vi "engine mappings UI.vi"() -> ()   [LabVIEW 2013, in "PL Framework Configuration Tool.lvlib" / "Engine Mappings.lvclass"]
uses:
  Engine Mappings.lvclass
  <vilib>/NI/CEF/CEF_TreeControl/Controls/EventCluster.ctl
  <vilib>/NI/CEF/CEF_TreeControl/NISE_CEF_TreeControl.lvlib
  <vilib>/NI/Module Execution Interface/Engine Configuration/engine configuration.lvclass
  <vilib>/NI/Tag Bus/tag/tag descriptor.lvclass
  Engine Parent/Engine Parent Editor Node.lvclass
  <vilib>/NI/CEF/CEF_TreeControl/Node/NodeRef.ctl
  <vilib>/NI/CEF/CEF_TreeControl/Node/NISE_CEF_Node.lvclass
  <vilib>/NI/Tools/Keyed Array/KeyedArray.ctl
  <vilib>/NI/Tools/Keyed Array/Tools_KeyedArray.lvlib
  <vilib>/NI/AMC/Message.ctl
  <vilib>/NI/AMC/AMC.lvlib
  <vilib>/NI/AMC/Message Queue.ctl
  <vilib>/NI/CEF/CEF_TreeControl/Node/UserEventRef.ctl
panel:
  in  "channels":i32(listbox)
  in  "main queue":T1
  in  "node ref":T2
  in  "Tags":i32(listbox)
  in  "user event":T3
  in  "unmap":bool
  in  "map":bool
  in  "Mappings":i32(listbox)
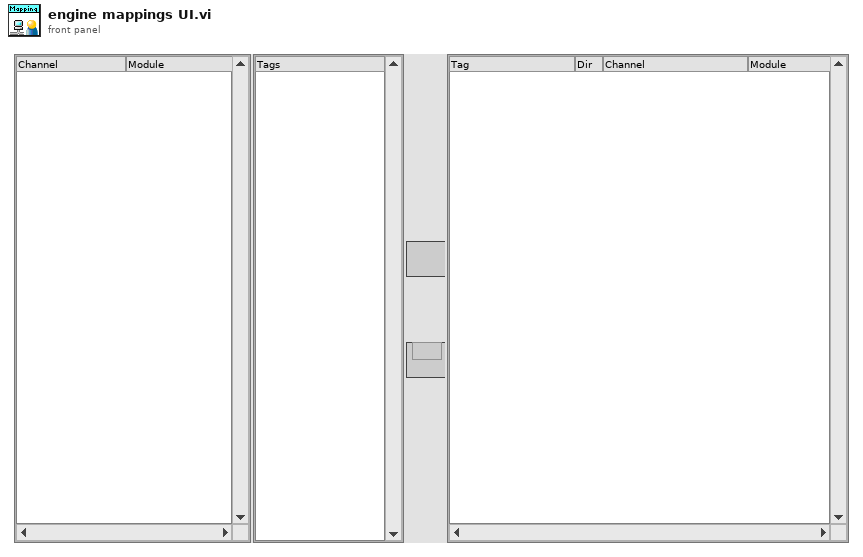
[diagram p1: front panel]
types:
  T1 = typedef "AMC.lvlib/Message Queue.ctl" = refnum<queue>
  T2 = typedef "NISE_CEF_Node.lvclass/NodeRef.ctl" = refnum<data-value>
  T3 = typedef "NISE_CEF_Node.lvclass/UserEventRef.ctl" = refnum<user-event>
  T4 = typedef "NISE_CEF_TreeControl.lvlib/EventCluster.ctl" = cluster{"command":string, "data":string}
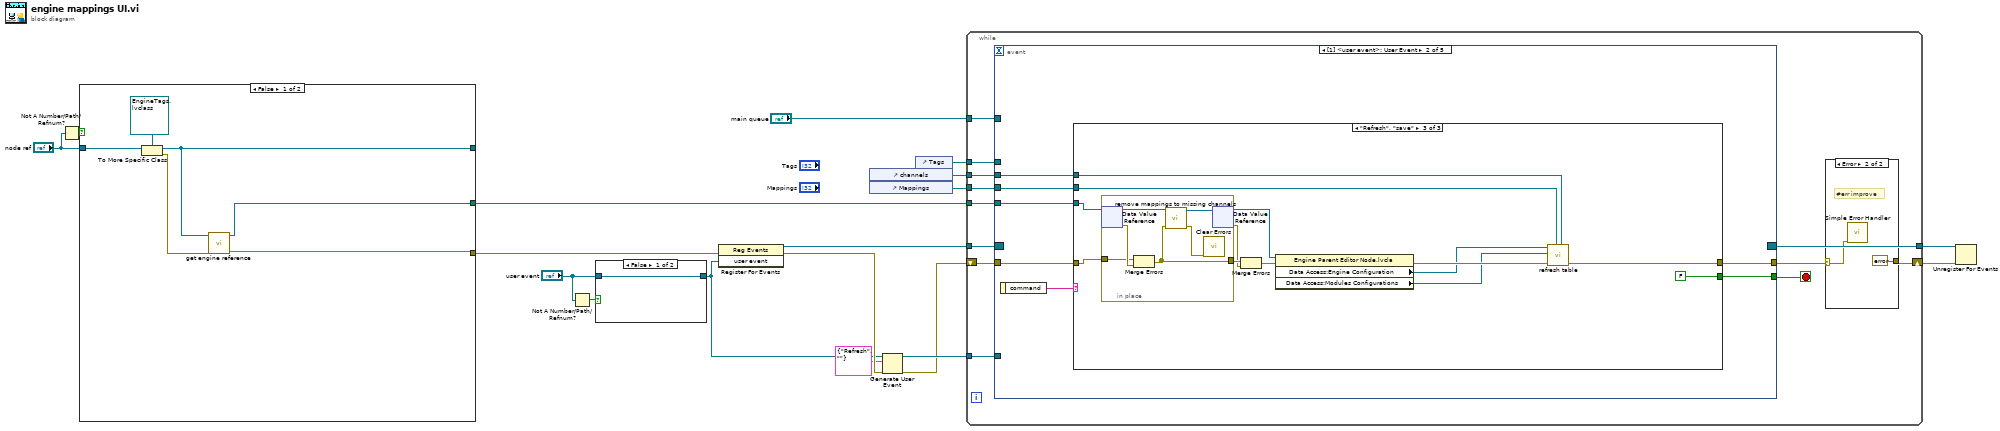
[diagram p0: block diagram]
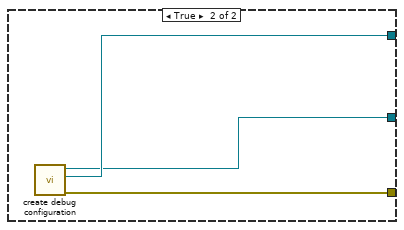
[diagram p2: hidden frame]
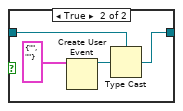
[diagram p3: hidden frame]
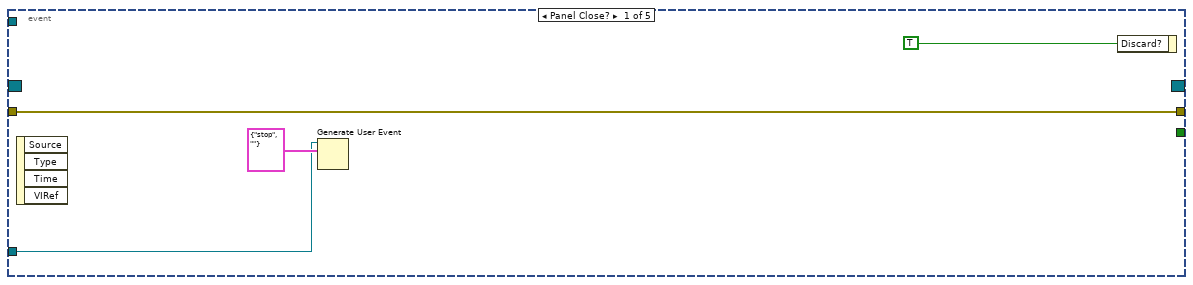
[diagram p5: hidden frame]
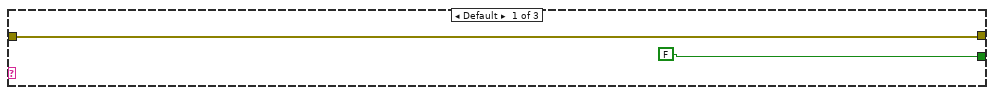
[diagram p6: hidden frame]
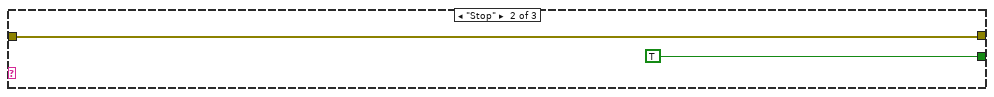
[diagram p7: hidden frame]
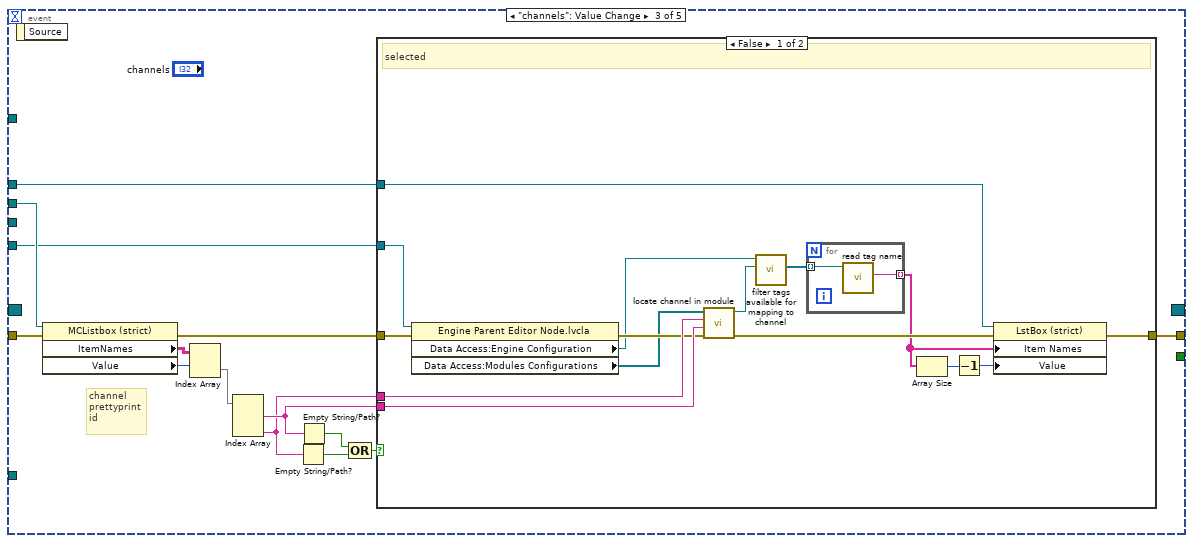
[diagram p8: hidden frame]
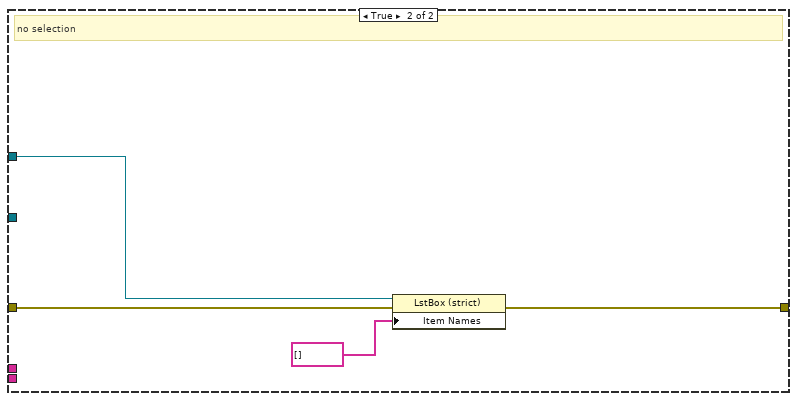
[diagram p9: hidden frame]
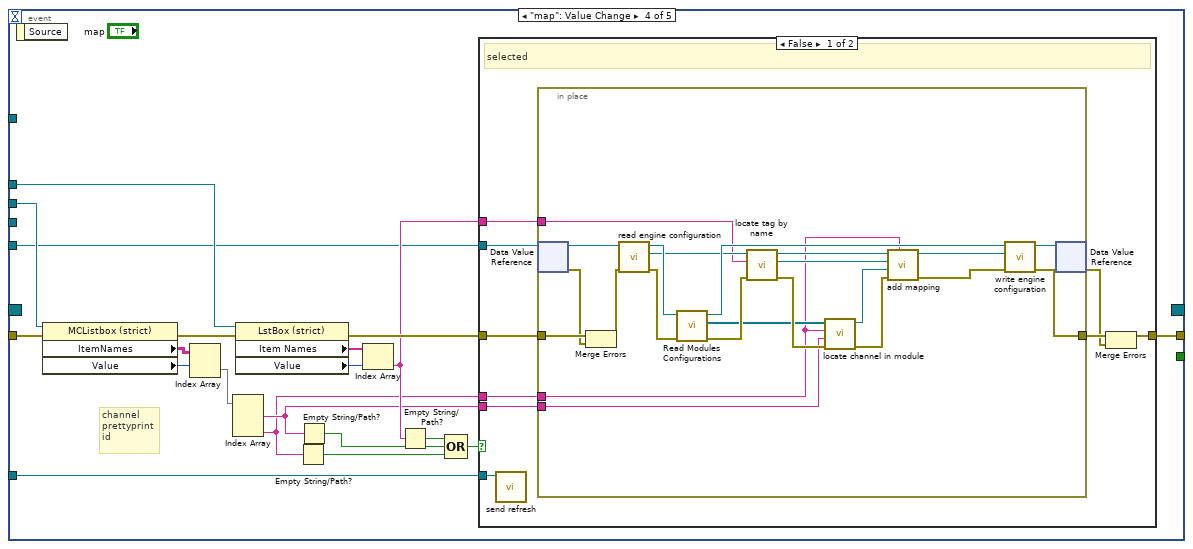
[diagram p10: hidden frame]
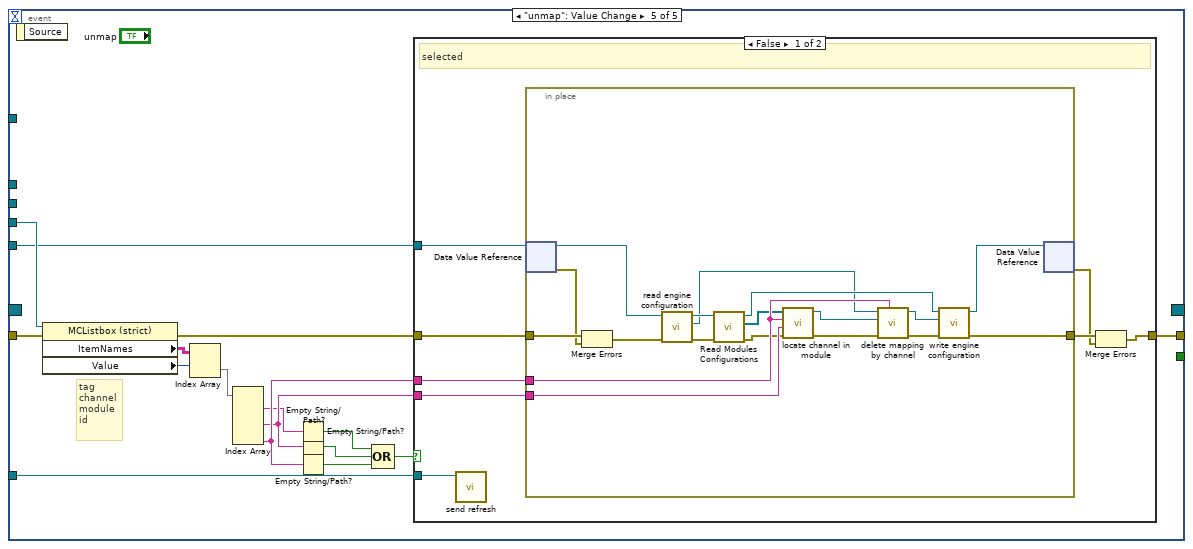
[diagram p12: hidden frame]
diagram:
  n1 = Not A Number/Path/Refnum?(number/path/refnum="node ref") -> (NaN/Path/Refnum?=w9:bool)
  n2 = case shown="False" w9 {
    tunnel: [w21 w27] -> _
    tunnel: [w22 w26] -> w1
    tunnel: [w20 w25] -> w13
    tunnel: "node ref" -> [w19 _]
    frame False {
      n3 = To More Specific Class(target class=refnum<data-value> refnum ("data value reference"), reference=w19) -> (specific class reference=w21:refnum<data-value>, error out=w23:errorcluster)  [unwired: 1 in]
      n4 = call "get engine reference.vi"("error in"=w23, "engine mappings"=w21) -> ("error out"=w22:errorcluster, "engine reference"=w20:refnum<data-value>)  [unwired: 8 in]
    }
    frame True {
      n5 = call "create debug configuration.vi"() -> ("error out"=w26:errorcluster, "mapping dvr"=w27:refnum<data-value>, "engine dvr"=w25:refnum<data-value>)  [unwired: 9 in]
    }
  }
  n6 = Not A Number/Path/Refnum?(number/path/refnum="user event") -> (NaN/Path/Refnum?=w11:bool)
  n7 = case shown="False" w11 {
    tunnel: [w28 w29] -> w8
    tunnel: "user event" -> [w28 w30]
    frame False {
    }
    frame True {
      n8 = Create User Event(user event datatype=T4 {"command"="", "data"=""} ("event data")) -> (user event=w31:refnum<user-event>)  [unwired: 1 in, 1 out]
      n9 = Type Cast(type=w30, x=w31) -> (*(type *) &x=w29:T3)
    }
  }
  n10 = register-events(error in=w1, w8) -> (reference out=w17:refnum<event-registration>, error out=w14:errorcluster)  [unwired: 1 in]
  n11 = control-ref of="channels"() -> (w3:refnum<vi>)
  n12 = control-ref of="Mappings"() -> (w2:refnum<vi>)
  n13 = Generate User Event(user event=w8, event data cluster=T4 {"command"="Refresh", "data"=""} ("event data"), error in=w14) -> (user event out=w7:T3, error out=w6:errorcluster)  [unwired: 1 in]
  n14 = control-ref of="Tags"() -> (w4:refnum<vi>)
  n15 = while {
    tunnel: "main queue" -> [w44]
    tunnel: w17 -> [w43]
    tunnel: [w42] -> w16
    shift-right: [w40] -> w15
    shift-left: w6 -> [w39]
    tunnel: w13 -> [w38]
    tunnel: w7 -> [w36]
    tunnel: w4 -> [w35]
    tunnel: w3 -> [w34]
    tunnel: w2 -> [w33]
    stop <- w41 stop-if-true
    n16 = event shown="[1] <user event>: User Event" {
      selector: w43 -> [_ _ _ _ _]
      dyn-events: [_ _ _ _ _] -> w42
      timeout: _ -> [_ _ _ _ _]
      tunnel: w44 -> [_ _ _ _ _]
      tunnel: [_ w55 _ _ _] -> w41
      tunnel: w39 -> [w51 w58 w95 w136 w184]
      tunnel: [w51 w57 w86 w122 w177] -> w37
      tunnel: w38 -> [_ w56 w82 w117 w169]
      tunnel: w36 -> [w49 _ _ w121 w176]
      tunnel: w35 -> [_ _ w83 w135 _]
      tunnel: w34 -> [_ w53 w93 w133 _]
      tunnel: w33 -> [_ w52 _ _ w175]
      event Panel Close? {
        n17 = event-data() -> ()  [unwired: 1 in, 4 out]
        n18 = Generate User Event(user event=w49, event data cluster=T4 {"command"="stop", "data"=""} ("event data")) -> ()  [unwired: 2 in, 2 out]
        n19 = event-data("Discard?"=TRUE) -> ()  [unwired: 1 in, 1 out]
      }
      event User Event {
        n20 = event-data() -> ("command"=w54:string)  [unwired: 1 in]
        n21 = case shown="\"Refresh\", \"save\"" w54 {
          tunnel: w58 -> [w60 w62 w66]
          tunnel: [w60 w62 w74] -> w57
          tunnel: w56 -> [_ _ w68]
          tunnel: [FALSE TRUE FALSE] -> w55
          tunnel: w53 -> [_ _ w73]
          tunnel: w52 -> [_ _ w72]
          frame Default {
          }
          frame "Stop" {
          }
          frame "Refresh", "save" {
            n22 = in-place {
              in-place-border: w66 -> [w80]
              in-place-border: [w77] -> w65
              n23 = in-place-dvr #1(w68) -> (w79:refnum<class "Engine Parent Editor Node.lvclass">, w81:errorcluster)
              n24 = Merge Errors(w80, w81) -> (w77:errorcluster)
              n25 = call "remove mappings to missing channels.vi"("error in"=w77, "Engine Parent Editor Node in"=w79) -> ("error out"=w76:errorcluster, "Engine Parent Editor Node out"=w78:refnum<class "Engine Parent Editor Node.lvclass">)  [unwired: 8 in]
              n26 = call <vilib>:"Clear Errors.vi"("error in (no error)"=w76) -> ()  [unwired: 6 in, 1 out]
              n27 = in-place-dvr #1(w78) -> (w67:refnum<data-value>, w64:errorcluster)
            }
            n28 = Merge Errors(w65, w64) -> (w63:errorcluster)
            n29 = property class="Engine Parent Editor Node.lvcla"(reference=w67, error in=w63) -> (error out=w71:errorcluster, "Data Access:Engine Configuration"=w70:refnum<class "engine configuration.lvclass">, "Data Access:Modules Configurations"=w69:refnum<class "TBM module configuration.lvclass">[])  [unwired: 1 out]
            n30 = call "refresh table.vi"("channels ref"=w73, "Mappings"=w72, "error in"=w71, "Modules Configurations"=w69, "engine configuration in"=w70) -> ("error out"=w74:errorcluster)  [unwired: 6 in]
          }
        }
      }
      event "channels": Value Change {
        # "channel\nprettyprint\nid"
        n31 = event-data() -> ()  [unwired: 1 in, 1 out]
        n32 = property class="MCListbox (strict)"(reference=w93, error in=w95) -> (error out=w94:errorcluster, "ItemNames"=w91:string[][], "Value"=w92:i32)  [unwired: 1 out]
        n33 = Index Array(array=w91, index (row)=w92) -> (element=w90:string[])  [unwired: 1 in]
        n34 = Index Array(array=w90) -> (element #1=w85:string, element #3=w84:string)  [unwired: 3 in, 1 out]
        n35 = Empty String/Path?(string/path=w84) -> (empty?=w89:bool)
        n36 = Empty String/Path?(string/path=w85) -> (empty?=w88:bool)
        n37 = Compound Arithmetic op=OR(w88, w89) -> (w87:bool)
        n38 = case shown="False" w87 {
          tunnel: w94 -> [w110 w116]
          tunnel: [w105 w115] -> w86
          tunnel: w85 -> [w109 _]
          tunnel: w84 -> [w108 _]
          tunnel: w83 -> [w106 w114]
          tunnel: w82 -> [w99 _]
          frame False {
            # "selected"
            n39 = property class="Engine Parent Editor Node.lvcla"(reference=w99, error in=w110) -> (error out=w98:errorcluster, "Data Access:Engine Configuration"=w96:refnum<class "engine configuration.lvclass">, "Data Access:Modules Configurations"=w97:refnum<class "TBM module configuration.lvclass">[])  [unwired: 1 out]
            n40 = call "locate channel in module.vi"("error in"=w98, "channel name"=w109, "instance id"=w108, "Modules Configurations"=w97) -> ("error out"=w104:errorcluster, "channel"=w107:refnum<class "TBM channel.lvclass">)  [unwired: 6 in]
            n41 = call <vilib>:"filter tags available for mapping to channel.vi"("channel to map to"=w107, "engine configuration in"=w96) -> ("filtered tags"=w103:refnum<class "tag descriptor.lvclass">[])  [unwired: 8 in, 1 out]
            n42 = for {
              tunnel: w103 -> [w112] mode=indexing
              tunnel: [w111] -> w102 mode=indexing
              n43 = call <vilib>:"read tag name.vi"("system tag in"=w112) -> ("name"=w111:string)  [unwired: 8 in, 2 out]
            }
            n44 = Array Size(array=w102) -> (size(s)=w101:i32)
            n45 = Decrement(x=w101) -> (x-1=w100:i32)
            n46 = property class="LstBox (strict)"(reference=w106, error in=w104, "Item Names"=w102, "Value"=w100) -> (error out=w105:errorcluster)  [unwired: 1 out]
          }
          frame True {
            # "no selection"
            n47 = property class="LstBox (strict)"(reference=w114, error in=w116, "Item Names"=string[] []) -> (error out=w115:errorcluster)  [unwired: 1 out]
          }
        }
      }
      event "map": Value Change {
        # "channel\nprettyprint\nid"
        n48 = event-data() -> ()  [unwired: 1 in, 1 out]
        n49 = property class="MCListbox (strict)"(reference=w133, error in=w136) -> (error out=w134:errorcluster, "ItemNames"=w131:string[][], "Value"=w132:i32)  [unwired: 1 out]
        n50 = Index Array(array=w131, index (row)=w132) -> (element=w128:string[])  [unwired: 1 in]
        n51 = Index Array(array=w128) -> (element #1=w119:string, element #3=w118:string)  [unwired: 3 in, 1 out]
        n52 = property class="LstBox (strict)"(reference=w135, error in=w134) -> (error out=w123:errorcluster, "Item Names"=w130:string[], "Value"=w129:i32)  [unwired: 1 out]
        n53 = Empty String/Path?(string/path=w118) -> (empty?=w127:bool)
        n54 = Empty String/Path?(string/path=w119) -> (empty?=w126:bool)
        n55 = Index Array(array=w130, index=w129) -> (element=w120:string)
        n56 = Empty String/Path?(string/path=w120) -> (empty?=w125:bool)
        n57 = Compound Arithmetic op=OR(w125, w126, w127) -> (w124:bool)
        n58 = case shown="False" w124 {
          tunnel: w123 -> [w144 w168]
          tunnel: [w142 w168] -> w122
          tunnel: w121 -> [w145 _]
          tunnel: w120 -> [w139 _]
          tunnel: w119 -> [w137 _]
          tunnel: w118 -> [w138 _]
          tunnel: w117 -> [w140 _]
          frame False {
            # "selected"
            n59 = call "send refresh.vi"("User Event in"=w145) -> ()  [unwired: 11 in]
            n60 = in-place {
              in-place-border: w144 -> [w167]
              in-place-border: [w162] -> w143
              in-place-border: w139 -> [w156]
              in-place-border: w138 -> [w146]
              in-place-border: w137 -> [w152]
              n61 = in-place-dvr #2(w140) -> (w159:refnum<class "Engine Parent Editor Node.lvclass">, w166:errorcluster)
              n62 = Merge Errors(w167, w166) -> (w165:errorcluster)
              n63 = call "read engine configuration.vi"("error in"=w165, "Engine Parent Editor Node in"=w159) -> ("error out"=w164:errorcluster, "engine configuration"=w158:refnum<class "engine configuration.lvclass">, "Engine Parent Editor Node out"=w163:refnum<class "Engine Parent Editor Node.lvclass">)  [unwired: 7 in]
              n64 = call "Read Modules Configurations.vi"("error in"=w164, "Engine Parent in"=w163) -> ("error out"=w155:errorcluster, "Component Configurations"=w153:refnum<class "TBM module configuration.lvclass">[], "Engine Parent out"=w160:refnum<class "Engine Parent Editor Node.lvclass">)  [unwired: 7 in]
              n65 = call <vilib>:"locate tag by name.vi"("error in"=w155, "tag name"=w156, "engine configuration in"=w158) -> ("error out"=w154:errorcluster, "tag descriptor"=w150:refnum<class "tag descriptor.lvclass">, "engine configuration out"=w157:refnum<class "engine configuration.lvclass">)  [unwired: 6 in]
              n66 = call "locate channel in module.vi"("error in"=w154, "channel name"=w152, "instance id"=w146, "Modules Configurations"=w153) -> ("error out"=w149:errorcluster, "channel"=w151:refnum<class "TBM channel.lvclass">)  [unwired: 6 in]
              n67 = call <vilib>:"add mapping.vi"("owner ID"=w146, "error in"=w149, "channel"=w151, "tag descriptor"=w150, "engine configuration"=w157) -> ("error out"=w148:errorcluster, "engine configuration out"=w147:refnum<class "engine configuration.lvclass">)  [unwired: 5 in]
              n68 = call "write engine configuration.vi"("error in"=w148, "engine configuration"=w147, "Engine Parent Editor Node in"=w160) -> ("error out"=w162:errorcluster, "Engine Parent Editor Node out"=w161:refnum<class "Engine Parent Editor Node.lvclass">)  [unwired: 7 in]
              n69 = in-place-dvr #2(w161) -> (w141:errorcluster)  [unwired: 1 out]
            }
            n70 = Merge Errors(w143, w141) -> (w142:errorcluster)
          }
          frame True {
            # "no selection"
          }
        }
      }
      event "unmap": Value Change {
        # "tag\nchannel\nmodule\nid"
        n71 = event-data() -> ()  [unwired: 1 in, 1 out]
        n72 = property class="MCListbox (strict)"(reference=w175, error in=w184) -> (error out=w183:errorcluster, "ItemNames"=w181:string[][], "Value"=w182:i32)  [unwired: 1 out]
        n73 = Index Array(array=w181, index (row)=w182) -> (element=w180:string[])  [unwired: 1 in]
        n74 = Index Array(array=w180) -> (element #1=w170:string, element #3=w171:string, element #5=w174:string)  [unwired: 5 in, 2 out]
        n75 = Empty String/Path?(string/path=w170) -> (empty?=w172:bool)
        n76 = Empty String/Path?(string/path=w171) -> (empty?=w173:bool)
        n77 = Empty String/Path?(string/path=w174) -> (empty?=w179:bool)
        n78 = Compound Arithmetic op=OR(w172, w173, w179) -> (w178:bool)
        n79 = case shown="False" w178 {
          tunnel: w183 -> [w191 w211]
          tunnel: [w186 w211] -> w177
          tunnel: w176 -> [w192 _]
          tunnel: w171 -> [w190 _]
          tunnel: w174 -> [w189 _]
          tunnel: w169 -> [w187 _]
          frame False {
            # "selected"
            n80 = call "send refresh.vi"("User Event in"=w192) -> ()  [unwired: 11 in]
            n81 = in-place {
              in-place-border: w191 -> [w210]
              in-place-border: w190 -> [w209]
              in-place-border: w189 -> [w206]
              in-place-border: [w198] -> w188
              n82 = in-place-dvr #3(w187) -> (w194:refnum<class "Engine Parent Editor Node.lvclass">, w205:errorcluster)
              n83 = Merge Errors(w210, w205) -> (w204:errorcluster)
              n84 = call "read engine configuration.vi"("error in"=w204, "Engine Parent Editor Node in"=w194) -> ("error out"=w203:errorcluster, "engine configuration"=w193:refnum<class "engine configuration.lvclass">, "Engine Parent Editor Node out"=w202:refnum<class "Engine Parent Editor Node.lvclass">)  [unwired: 7 in]
              n85 = call "Read Modules Configurations.vi"("error in"=w203, "Engine Parent in"=w202) -> ("error out"=w201:errorcluster, "Component Configurations"=w200:refnum<class "TBM module configuration.lvclass">[], "Engine Parent out"=w195:refnum<class "Engine Parent Editor Node.lvclass">)  [unwired: 7 in]
              n86 = call "locate channel in module.vi"("error in"=w201, "channel name"=w209, "instance id"=w206, "Modules Configurations"=w200) -> ("error out"=w208:errorcluster, "channel"=w207:refnum<class "TBM channel.lvclass">)  [unwired: 6 in]
              n87 = call <vilib>:"delete mapping by channel.vi"("owner ID"=w206, "error in"=w208, "channel"=w207, "engine configuration in"=w193) -> ("error out"=w199:errorcluster, "engine configuration out"=w196:refnum<class "engine configuration.lvclass">)  [unwired: 6 in]
              n88 = call "write engine configuration.vi"("error in"=w199, "engine configuration"=w196, "Engine Parent Editor Node in"=w195) -> ("error out"=w198:errorcluster, "Engine Parent Editor Node out"=w197:refnum<class "Engine Parent Editor Node.lvclass">)  [unwired: 7 in]
              n89 = in-place-dvr #3(w197) -> (w185:errorcluster)  [unwired: 1 out]
            }
            n90 = Merge Errors(w188, w185) -> (w186:errorcluster)
          }
          frame True {
            # "no selection"
          }
        }
      }
    }
    n91 = case shown="Error" w37 {
      selector: w37 -> [w45 w47]
      tunnel: [w45 errorcluster {"status"=FALSE, "code"=0, "source"=""} ("error IO")] -> w40
      frame No Error {
      }
      frame Error {
        # "#err improve"
        n92 = call <vilib>:"Simple Error Handler.vi"("error in (no error)"=w47) -> ()  [unwired: 4 in, 5 out]
      }
    }
  }
  n93 = Unregister For Events(event registration refnum=w16, error in=w15) -> ()  [unwired: 1 out]
